vi "Intake_Begin.vi"   [LabVIEW 2019]
uses:
  Intake_Cluster.ctl
  Intake_States.ctl
  Intake_Globals.vi
types:
  T1 = typedef "Intake_Cluster.ctl" = cluster{"Control_State":T2, "Intake_On":bool, "Intake_Extended":bool, "Intake_Throttle":dbl, "Auto_Notifier":refnum<notifier>, "Parameter_1":dbl, "Parameter_2":dbl, "Step":dbl, "Outtake":bool}
  T2 = typedef "Intake_States.ctl" = enum16{"Manual_Throttle", "Manual_Single_Speed", "Compliant_Intake", "Command_RunIntake"}
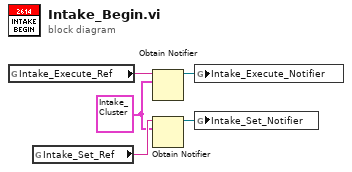
[diagram p0: block diagram]
diagram:
  w3 = T1 {"Control_State"=enum."Manual_Throttle", "Intake_On"=FALSE, "Intake_Extended"=FALSE, "Intake_Throttle"=0.0, "Auto_Notifier"=refnum, "Parameter_1"=0.0, "Parameter_2"=0.0, "Step"=0.0, "Outtake"=FALSE} ("Intake_Cluster")
  n1 = global read "Intake_Globals.vi" "Intake_Execute_Ref"() -> (w4:string)
  n2 = global read "Intake_Globals.vi" "Intake_Set_Ref"() -> (w5:string)
  n3 = Obtain Notifier(name (unnamed)=w4, notification data type=w3) -> (notifier out=w2:refnum<notifier>)  [unwired: 2 in, 2 out]
  n4 = Obtain Notifier(name (unnamed)=w5, notification data type=w3) -> (notifier out=w1:refnum<notifier>)  [unwired: 2 in, 2 out]
  n5 = global write "Intake_Globals.vi" "Intake_Execute_Notifier"(w2) -> ()
  n6 = global write "Intake_Globals.vi" "Intake_Set_Notifier"(w1) -> ()
